vi "EndTest.vi"(7 "Time":dbl, 8 "error in (no error)":errorcluster, 10 "TestCase":refnum<class "TestCase.lvclass">, 11 "EventTestListener in":refnum<class "EventTestListener.lvclass">) -> (0 "error out":errorcluster, 3 "EventTestListener out":refnum<class "EventTestListener.lvclass">)   [LabVIEW 2019, in "TestExplorer.lvlib" / "EventTestListener.lvclass"]
doc: "A test ended."
uses:
  EventTestListener.lvclass
  TestCase/TestCase/TestCase.lvclass
  TestEndedEventData.ctl
  EventTestListener.lvclass/EventTestListener.ctl
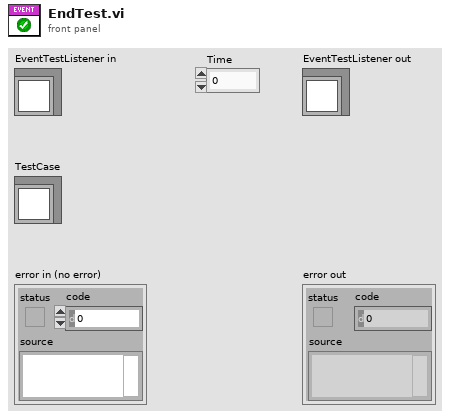
[diagram p1: front panel]
types:
  T1 = typedef "TestExplorer.lvlib/EventTestListener.lvclass/TestEndedEventData.ctl" = cluster{"TestCase":refnum<class "TestCase.lvclass">, "Time":dbl}
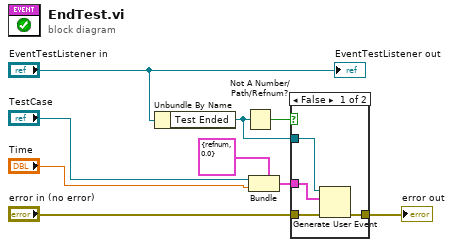
[diagram p0: block diagram]
diagram:
  n1 = Unbundle By Name("EventTestListener in") -> ("Test Ended"=w2:refnum<user-event>)
  n2 = Not A Number/Path/Refnum?(number/path/refnum=w2) -> (NaN/Path/Refnum?=w1:bool)
  n3 = Bundle(cluster=T1 {"TestCase"=refnum, "Time"=0.0} ("FailureEventData"), "TestCase"="TestCase", "Time"="Time") -> (w4:T1)
  n4 = case shown="False" w1 {
    tunnel: "error in (no error)" -> [w13 w14]
    tunnel: [w12 w14] -> w8
    tunnel: w2 -> [w11 _]
    tunnel: w4 -> [w10 _]
    frame False {
      n5 = Generate User Event(user event=w11, event data cluster=w10, error in=w13) -> (error out=w12:errorcluster)  [unwired: 1 in, 1 out]
    }
    frame True {
    }
  }
  "error out" <- w8
  "EventTestListener out" <- "EventTestListener in"
